vi "ClusterToAttrMap.vi"(8 "error in (no error)":errorcluster, 11 "data":variant) -> (0 "error out":errorcluster, 3 "AttrMap":T1)   [LabVIEW 2019, in "lv-apt-json-file.lvlib"]
uses:
  <userlib>/_lvAPT/lv-apt-json-file/lv-apt-json-file.lvlib
  <userlib>/_lvAPT/lv-apt-json-file/Typedef/Def-AttrMap.ctl
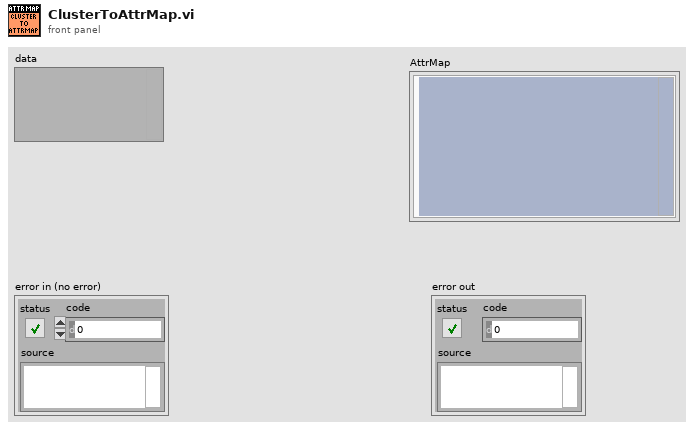
[diagram p1: front panel]
types:
  T1 = typedef "lv-apt-json-file.lvlib/Def-AttrMap.ctl" = cluster{"Map":variant}
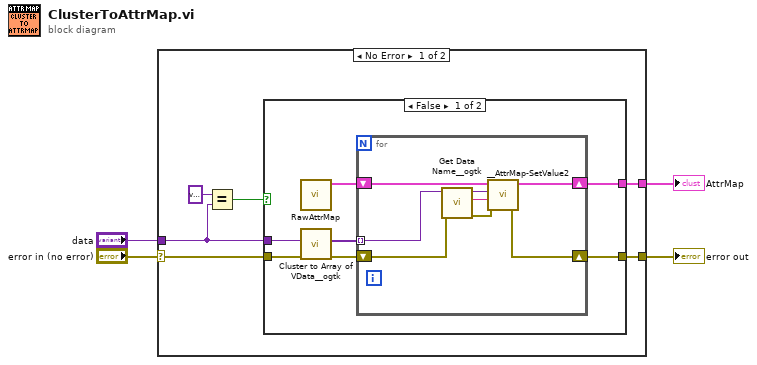
[diagram p0: block diagram]
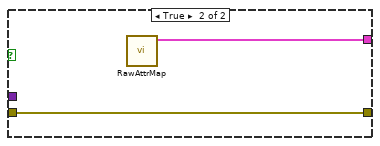
[diagram p2: hidden frame]
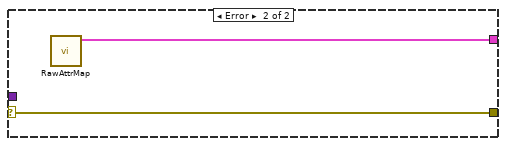
[diagram p3: hidden frame]
diagram:
  n1 = case shown="No Error" "error in (no error)" {
    selector: "error in (no error)" -> [w8 w29]
    tunnel: [w10 w28] -> w4
    tunnel: [w9 w29] -> w3
    tunnel: "data" -> [w6 _]
    frame No Error {
      n2 = Equal?(x=variant, y=w6) -> (x = y?=w5:bool)
      n3 = case shown="False" w5 {
        tunnel: [w17 w26] -> w10
        tunnel: [w16 w27] -> w9
        tunnel: w8 -> [w15 w27]
        tunnel: w6 -> [w12 _]
        frame False {
          n4 = call <userlib>:"RawAttrMap.vi"() -> ("AttrMap"=w11:T1)  [unwired: 11 in]
          n5 = call <userlib>:"Cluster to Array of VData__ogtk.vi"("error in (no error)"=w15, "Cluster"=w12) -> ("error out"=w14:errorcluster, "Array of VData"=w13:variant[])  [unwired: 8 in]
          n6 = for {
            tunnel: w13 -> [w24] mode=indexing
            shift-right: [w22] -> w17
            shift-left: w11 -> [w23]
            shift-right: [w21] -> w16
            shift-left: w14 -> [w25]
            n7 = call <userlib>:"Get Data Name__ogtk.vi"("error in (no error)"=w25, "Data"=w24) -> ("error out"=w20:errorcluster, "Data Name"=w18:string, "Data dup"=w19:variant)  [unwired: 7 in]
            n8 = call <userlib>:"__AttrMap-SetValue2.vi"("error in (no error)"=w20, "Key"=w18, "Value"=w19, "AttrMap in"=w23) -> ("error out"=w21:errorcluster, "AttrMap out"=w22:T1)  [unwired: 6 in]
          }
        }
        frame True {
          n9 = call <userlib>:"RawAttrMap.vi"() -> ("AttrMap"=w26:T1)  [unwired: 11 in]
        }
      }
    }
    frame Error {
      n10 = call <userlib>:"RawAttrMap.vi"() -> ("AttrMap"=w28:T1)  [unwired: 11 in]
    }
  }
  "AttrMap" <- w4
  "error out" <- w3
